vi "to string.vi"(8 "error in":errorcluster, 11 "TEC configuration in":refnum<class "TEC configuration.lvclass">) -> (0 "error out":errorcluster, 1 "data":string, 2 "version":string, 3 "TEC configuration out":refnum<class "TEC configuration.lvclass">)   [LabVIEW 2013, in "TEC configuration.lvclass"]
doc: "Provides an interface for saving a module configuration to a file or other serialized data source. It is recommended that all children of this class store data in two sets--data required for its own initialization, and any data required for parent initialization--and that each implementation uses the <b>Call Parent Method</b> primitive to serialize parent information."
uses:
  TEC configuration.lvclass
  <vilib>/NI/Tag Bus Module Framework/module configuration/TBM module configuration.lvclass
  TEC configuration.lvclass/TEC configuration.ctl
  <vilib>/NI/Tag Bus Module Framework/root configuration/unwrap data.vi
  <vilib>/NI/Tag Bus Module Framework/root configuration/TBM configuration.lvclass
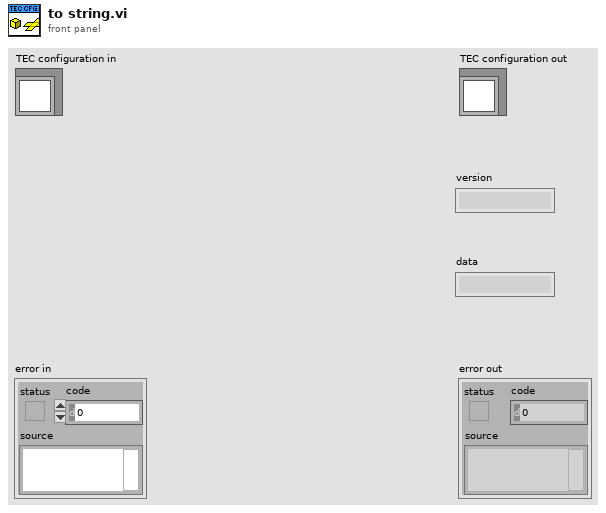
[diagram p1: front panel]
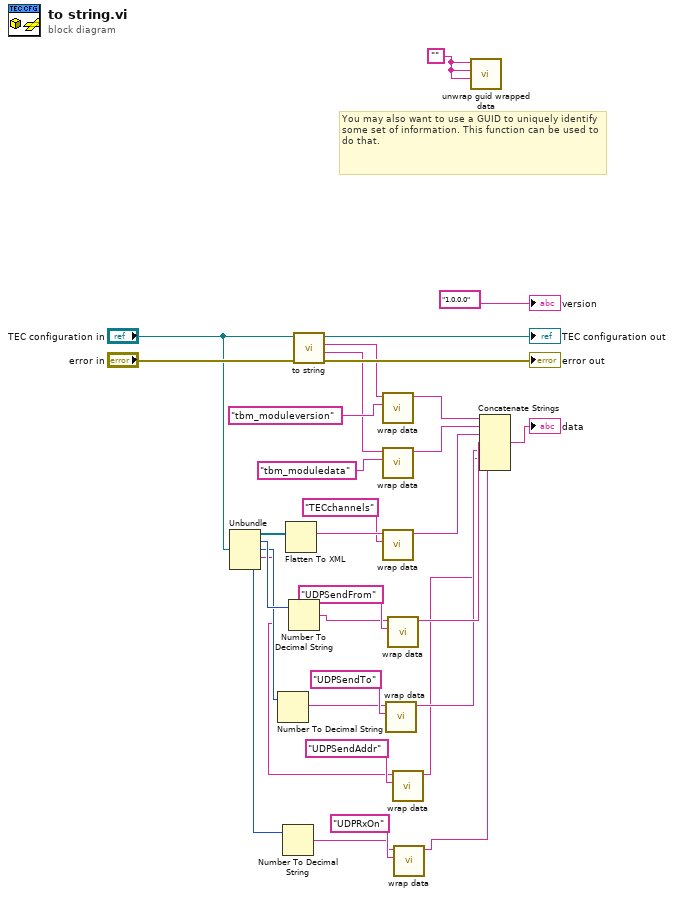
[diagram p0: block diagram]
diagram:
  w23 = ""
  # "You may also want to use a GUID to uniquely identify some set of information. This function can be used to do that."
  n1 = Unbundle("TEC configuration in") -> (w20:refnum<class "TBM channel.lvclass">[], w7:u16, w4:u16, w3:string, w2:u16)
  n2 = Number To Decimal String(number=w4) -> (decimal integer string=w5:string)  [unwired: 1 in]
  n3 = Number To Decimal String(number=w2) -> (decimal integer string=w1:string)  [unwired: 1 in]
  n4 = Flatten To XML(anything=w20) -> (xml string=w19:string)
  n5 = Number To Decimal String(number=w7) -> (decimal integer string=w6:string)  [unwired: 1 in]
  n6 = call-parent "to string.vi"("error in"="error in", "module configuration in"="TEC configuration in") -> ("error out"=→"error out":errorcluster, "data"=w24:string, "version"=w25:string, "module configuration out"=→"TEC configuration out":refnum<class "TEC configuration.lvclass">)  [unwired: 6 in]
  n7 = call <vilib>:"wrap data.vi"("identifier"="tbm_moduleversion" ("additional identifier"), "data to wrap"=w25) -> ("wrapped data"=w27:string)  [unwired: 9 in]
  n8 = call <vilib>:"wrap data.vi"("identifier"="tbm_moduledata" ("additional identifier"), "data to wrap"=w24) -> ("wrapped data"=w26:string)  [unwired: 9 in]
  n9 = call <vilib>:"wrap data.vi"("identifier"="TECchannels" ("additional identifier"), "data to wrap"=w19) -> ("wrapped data"=w18:string)  [unwired: 9 in]
  n10 = call <vilib>:"wrap data.vi"("identifier"="UDPSendTo" ("additional identifier"), "data to wrap"=w5) -> ("wrapped data"=w10:string)  [unwired: 9 in]
  n11 = call <vilib>:"wrap data.vi"("identifier"="UDPSendFrom" ("additional identifier"), "data to wrap"=w6) -> ("wrapped data"=w11:string)  [unwired: 9 in]
  n12 = call <vilib>:"wrap data.vi"("identifier"="UDPSendAddr" ("additional identifier"), "data to wrap"=w3) -> ("wrapped data"=w9:string)  [unwired: 9 in]
  n13 = call <vilib>:"wrap data.vi"("identifier"="UDPRxOn" ("additional identifier"), "data to wrap"=w1) -> ("wrapped data"=w8:string)  [unwired: 9 in]
  n14 = call <vilib>:"unwrap guid wrapped data.vi"("identifier"=w23, "uuid"=w23, "data to unwrap"=w23) -> ()  [unwired: 7 in, 2 out]
  n15 = Concatenate Strings(w27, w26, w18, w11, w10, w9, w8) -> (→"data":string)
  "version" <- "1.0.0.0" ("current version")
